vi "RSZVB Set Trace Compression Value.vi"(8 "error in (no error)":errorcluster {"code" format="%.0x"}, 9 "Compression Value (1.0 dBm)":dbl=1.0 format="%^.3e", 10 "Channel (Trace) (1)":i32=1, 11 "VISA session":refnum<visa-resource-name>) -> (0 "error out":errorcluster {"code" format="%.0x"}, 3 "dup VISA session":refnum<visa-resource-name>)   [LabVIEW 2011]
doc: "This VI defines the compression value x for the x-dB compression point measurement.\n\nRemote-control command(s):\nCALCulate<Chn>:STATistics:NLINear:COMP:LEVel"
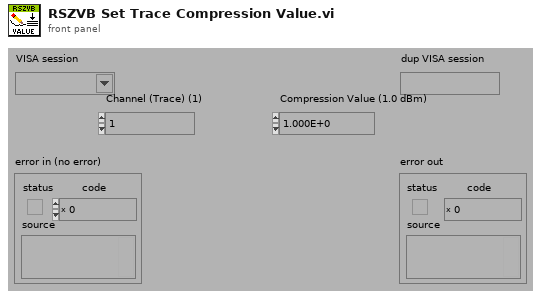
[diagram p1: front panel]
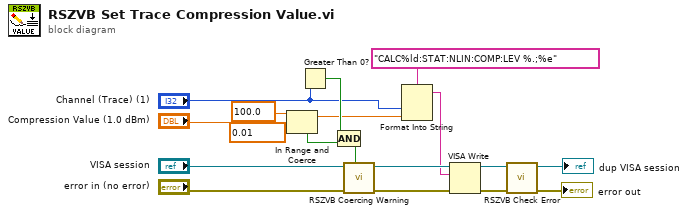
[diagram p0: block diagram]
diagram:
  n1 = In Range and Coerce(upper limit=100.0, x="Compression Value (1.0 dBm)", lower limit=0.01) -> (coerced(x)=w7:dbl, In Range?=w8:bool)
  n2 = Greater Than 0?(x="Channel (Trace) (1)") -> (x > 0?=w11:bool)
  n3 = Compound Arithmetic op=AND(w11, w8) -> (w13:bool)
  n4 = call "RSZVB Coercing Warning.vi"("In Range?"=w13, "error in (no error)"="error in (no error)", "VISA session"="VISA session") -> ("error out"=w16:errorcluster, "dup VISA session"=w17:refnum<visa-resource-name>)  [unwired: 7 in]
  n5 = Format Into String(format string="CALC%ld:STAT:NLIN:COMP:LEV %.;%e", "Channel (Trace) (1)", w7) -> (resulting string=w12:string)  [unwired: 2 in, 1 out]
  n6 = VISA Write(VISA resource name=w17, write buffer=w12, error in (no error)=w16) -> (VISA resource name out=w14:refnum<visa-resource-name>, error out=w15:errorcluster)  [unwired: 1 out]
  n7 = call "RSZVB Check Error.vi"("error in (no error)"=w15, "VISA session"=w14) -> ("error out"=→"error out":errorcluster, "dup VISA session"=→"dup VISA session":refnum<visa-resource-name>)  [unwired: 8 in]
